vi "niRFUtil RFHS Benchmark Create.vi"(0 "Task Name":string, 1 "Reset Database":bool, 5 "Buffer Size":u32=2048, 11 "error in (no error)":errorcluster) -> (4 "BenchmarkTask":T1, 6 "Frequency":u64, 15 "error out":errorcluster)   [LabVIEW 2015, in "niRFUtil.lvlib"]
uses:
  niRFUtil.lvlib
  niRFUtil RFHS Benchmark Task.ctl
  niRFUtil RFHS Util Phases.ctl
  kernel32.dll
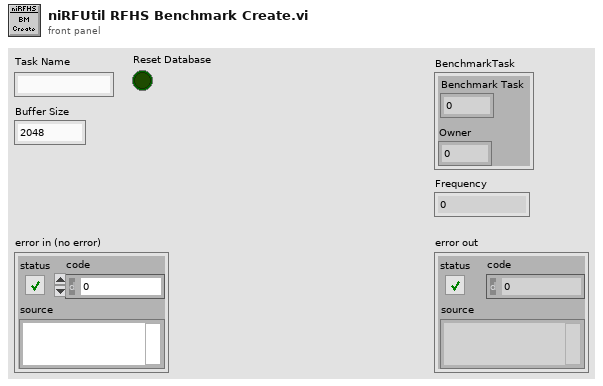
[diagram p1: front panel]
types:
  T1 = typedef "niRFUtil.lvlib/niRFUtil RFHS Benchmark Task.ctl" = cluster{"Benchmark Task":u64, "Owner":u32}
  T2 = typedef "niRFUtil.lvlib/niRFUtil RFHS Util Phases.ctl" = enum32{"Reserved", "CreateBenchmarkTask", "CRC", "UE UL Segment Transport Block", "UE UL Read Buffer", "UE UL TC", "UE UL RM", "UE UL CI", "Scramble", "Group Bits", "Benchmark Task Start", "Benchmark Task Stop", "Descramble", "Deinterleave", "eNB UL HARQ", "eNB UL Read Buffer", "eNB UL AFEM", "eNB UL Turbo Decoder", "Get Benchmark Task Data", "G31", "UL Gen Freq2Time", "Gen Power Spectrum", "UL Ana Time2Freq", "Benchmark Task Enter", "Benchmark Task Leave"}
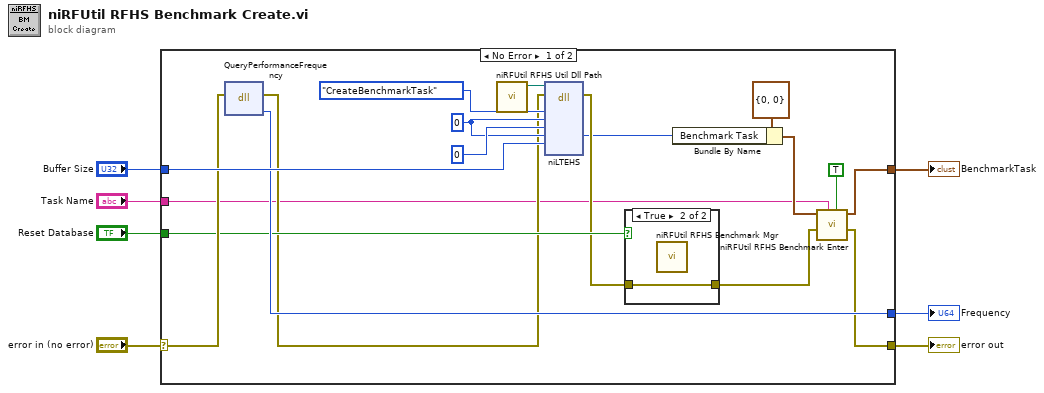
[diagram p0: block diagram]
diagram:
  n1 = case shown="No Error" "error in (no error)" {
    selector: "error in (no error)" -> [w20 w28]
    tunnel: [w9 w28] -> w2
    tunnel: "Buffer Size" -> [w21 _]
    tunnel: [w19 _] -> w4
    tunnel: "Reset Database" -> [w18 _]
    tunnel: "Task Name" -> [w11 _]
    tunnel: [w8 _] -> w1
    frame No Error {
      w22 = u64 0 ("benchmarkTask")
      n2 = dll-call lib="kernel32.dll" fn="QueryPerformanceFrequency"(error in=w20) -> (error out=w17:errorcluster, "frequency"=w19:u64)  [unwired: 4 in, 1 out]
      n3 = call "niRFUtil RFHS Util Dll Path.vi"() -> ("Path"=w25:path)  [unwired: 7 in, 4 out]
      n4 = dll-call lib="C:/ni-rt/system/HPCExecBenchDll.dll" fn="niLTEHS"(path in=w25, error in=w17, "what"=niRFUtil_RFHS_Util_Phases."CreateBenchmarkTask" ("Enum"), "benchmarkTask"=w22, "benchId"=u32 0, "newBenchmarkTask"=w22, "bufferSize"=w21) -> (error out=w16:errorcluster, "newBenchmarkTask"=w12:u64)  [unwired: 8 in, 1 out]
      n5 = case shown="True" w18 {
        tunnel: [w26 w27] -> w10
        tunnel: w16 -> [w26 w27]
        frame False {
        }
        frame True {
          n6 = call "niRFUtil RFHS Benchmark Mgr.vi"() -> ()  [unwired: 14 in, 2 out]
        }
      }
      n7 = Bundle By Name(cluster=T1 {"Benchmark Task"=0, "Owner"=0} ("BenchmarkTask"), "Benchmark Task"=w12) -> (w14:T1)
      n8 = call "niRFUtil RFHS Benchmark Enter.vi"("ID Changed"=TRUE, "ID"=w11, "error in (no error)"=w10, "Benchmark Task (Parent)"=w14) -> ("error out"=w9:errorcluster, "Benchmark Task (Self)"=w8:T1)  [unwired: 6 in]
    }
    frame Error {
    }
  }
  "error out" <- w2
  "BenchmarkTask" <- w1
  "Frequency" <- w4
